vi "gui.vi"() -> ()   [LabVIEW 2026]
uses:
  <vilib>/Instr/_visa.llb/VISA Configure Serial Port (Instr).vi
panel:
  in  "RST":bool caption="Boolean"
  out "Today":timestamp format="%<%X\n%x>T"
  out "Servo Angle":dbl(graph)
  out "Buzzer Volume":dbl(graph)
  out "Reset to\nOpen?":bool
  out "Force\nClose?":bool
  out "Rain \nDetected?":bool
  out "Physical Switch State (D)":dbl
  out "RSM (Digital)":dbl
  out "Buzzer Volume (A)":dbl
  out "RSM (Analog)":dbl
  out "Servo Angle (A)":dbl
  out "Raw Data":string
  in  "stop":bool
  out "Rain Intensity":dbl(slide) scale=0.0..100.0
  in  "Select Serial Port":refnum<visa-resource-name>="ASRL5::INSTR"
  # "EMBEDDED RAIN RESPONSIVE\n  SERVO CONTROL SYSTEM\n       By Group 03\n  (CPE109L-4 B1 2T2526) \n          Acot, Jose Julian\n          Bendol, Cherry Ben Jr.\n          Padilla, Kristian Emmanuel"
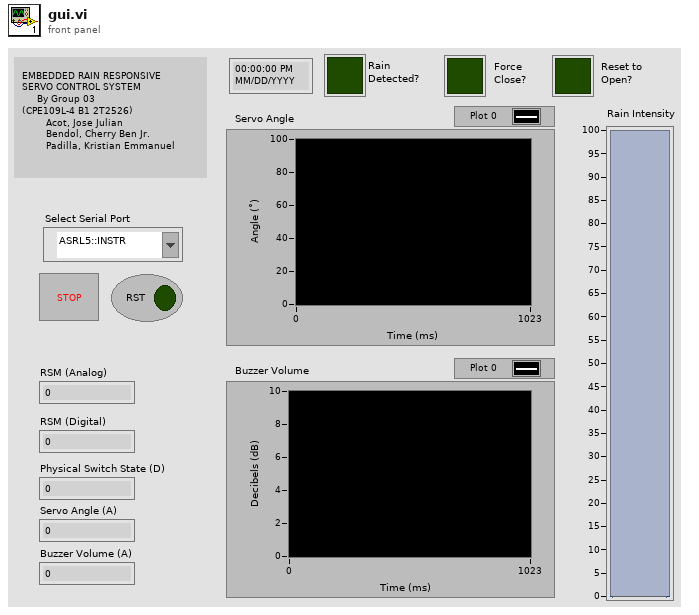
[diagram p1: front panel]
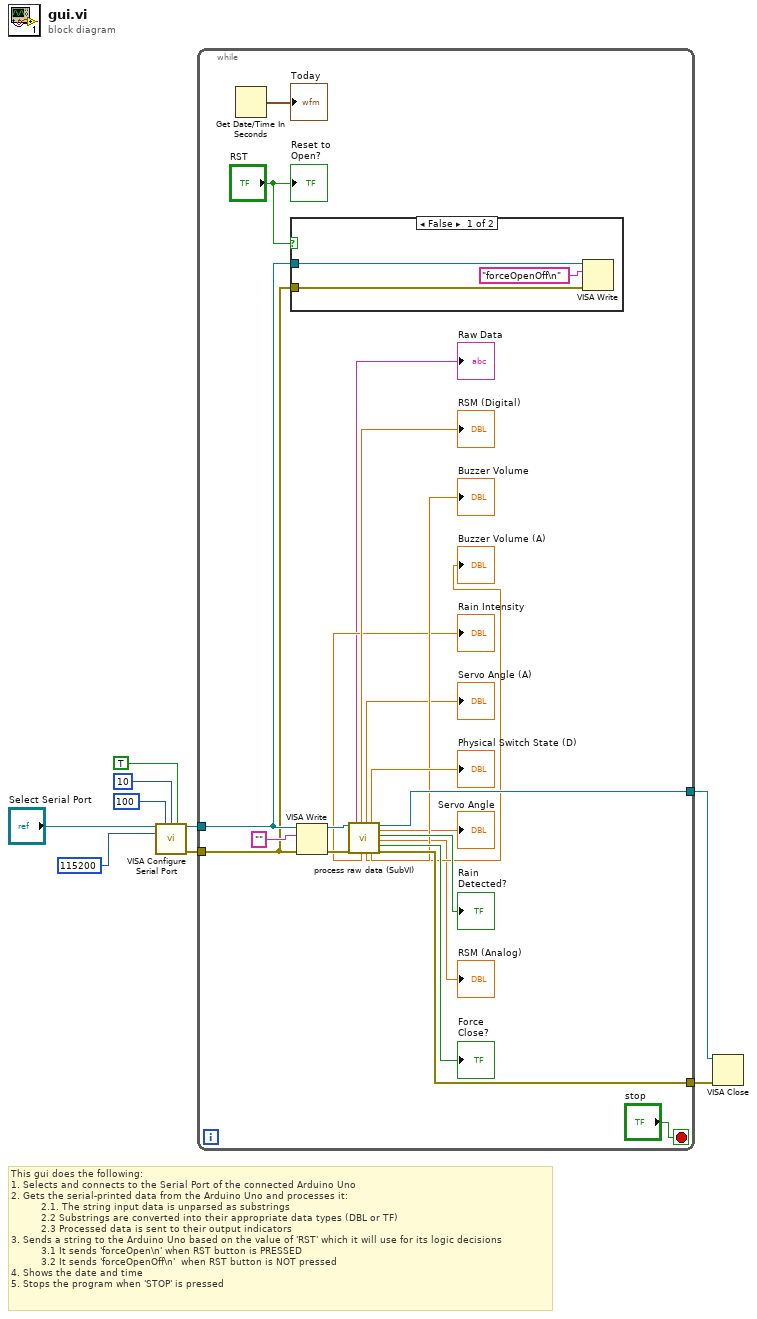
[diagram p0: block diagram]
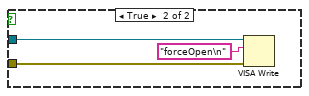
[diagram p2: hidden frame]
diagram:
  # "This gui does the following:\n1. Selects and connects to the Serial Port of the connected Arduino Uno\n2. Gets the serial-printed data from the Arduino Uno and processes it:\n          2.1. The string input data is unparsed as substrings\n          2.2 Substrings are converted into their appropriate data types (DBL or TF)\n          2.3 Processed data is sent to their output indicators\n3. Sends a string to the Arduino Uno based on the value of 'RST' which it will use for its logic decisions\n          3.1 It sends 'forceOpen\\n' when RST button is PRESSED\n          3.2 It sends 'forceOpenOff\\n'  when RST button is NOT pressed\n4. Shows the date and time \n5. Stops the program when 'STOP' is pressed"
  n1 = call-poly "VISA Configure Serial Port"("VISA resource name"="Select Serial Port", "timeout (10sec)"=u32 100, "termination char\n(0xA = '\\n' = LF)"=u8 10 ("termination char\n(0xA = '\\n' = LF)"), "Enable Termination\nChar (T)"=TRUE ("Enable Termination\nChar (T)"), "baud rate (9600)"=u32 115200) -> ("VISA resource name out"=w8:refnum<visa-resource-name>, "error out"=w7:errorcluster)  [unwired: 9 in]
  n2 = while {
    tunnel: w8 -> [w12]
    tunnel: w7 -> [w11]
    tunnel: [w30] -> w6
    tunnel: [w29] -> w5
    stop <- "stop" stop-if-true
    n3 = Get Date/Time In Seconds() -> (seconds since 1Jan1904=→"Today":timestamp)
    n4 = case shown="False" "RST" {
      tunnel: w12 -> [w32 w35]
      tunnel: w11 -> [w31 w34]
      frame False {
        n5 = VISA Write(VISA resource name=w32, write buffer="forceOpenOff\n", error in (no error)=w31) -> ()  [unwired: 3 out]
      }
      frame True {
        n6 = VISA Write(VISA resource name=w35, write buffer="forceOpen\n", error in (no error)=w34) -> ()  [unwired: 3 out]
      }
    }
    n7 = VISA Write(VISA resource name=w12, write buffer="", error in (no error)=w11) -> (VISA resource name out=w25:refnum<visa-resource-name>, error out=w26:errorcluster)  [unwired: 1 out]
    n8 = call "process raw data (SubVI).vi"("VISA Refnum in"=w25, "error in (no error)"=w26) -> ("Raw Data"=→"Raw Data":string, "RSM (Digital)"=→"RSM (Digital)":dbl, "Rain Intensity"=→"Rain Intensity":dbl, "Servo Angle (A)"=→"Servo Angle (A)":dbl, "Buzzer Volume (A)"=→"Buzzer Volume (A)":dbl, "Physical Switch State (D)"=→"Physical Switch State (D)":dbl, "Buzzer Volume"=→"Buzzer Volume":dbl, "VISA Refnum out"=w30:refnum<visa-resource-name>, "Servo Angle"=→"Servo Angle":dbl, "Rain \nDetected?"=→"Rain \nDetected?":bool, "RSM (Analog)"=→"RSM (Analog)":dbl, "Force\nClose?"=→"Force\nClose?":bool, "error out"=w29:errorcluster)  [unwired: 5 in]
    "Reset to\nOpen?" <- "RST"
  }
  n9 = VISA Close(VISA resource name=w6, error in (no error)=w5) -> ()  [unwired: 1 out]
